vi "Billard2020.vi"(11 "Path":path) -> (0 "Error out":errorcluster)   [LabVIEW 2019]
doc: "Billard2020.vi\n-Call Get_Box or Get_Box_No_Loop, then Call_C, then Draw_Line, then Save_to_Matlab and finally run Analyse.m. \n-To run this VI you have to provide the path of the desired sequence.\n-You can choose before runing if you want to create a ScoreSheet.\n-You can also personalize ScoreSheet.pdf with Band Touch, Ball Touch and Line (as described in the context help of Save_to_Matlab) and choose the detection method of the Billard box (with or without loop).\n-If an error occurs you can get more information about the error by consulting the PDF docsumentation or on : \nhttp://zone.ni.com/reference/fr-XX/help/371361R-0114/lverror/misc_lv_error_codes/"
panel:
  in  "Dark Blue Frame":T1={"Rmax"=14.0, "Rmin"=0.0, "Gmax"=42.0, "Gmin"=0.0, "Bmax"=126.0, "Bmin"=121.0}
  in  "Get Box Whithout Loop":bool
  in  "Parameters":T2={"RedBall"={"Rmin"=160.0, "Rmax"=255.0, "Gmin"=0.0, "Gmax"=160.0, "Bmin"=0.0, "Bmax"=160.0}, "YellowBall"={"Rmin"=140.0, "Rmax"=255.0, "Gmin"=140.0, "Gmax"=255.0, "Bmin"=0.0, "Bmax"=175.0}, "WhiteBall"={"Rmin"=100.0, "Rmax"=255.0, "Gmin"=100.0, "Gmax"=255.0, "Bmin"=100.0, "Bmax"=255.0}, "BlueBG"={"Rmin"=39.0, "Rmax"=62.0, "Gmin"=91.0, "Gmax"=116.0, "Bmin"=202.0, "Bmax"=255.0}, "BallDiameter"=11.0}
  in  "Line":string=".-"
  in  "Ball Touch":u32(colorbox)=1238015
  in  "Band Touch":u32(colorbox)=6618880
  in  "Create Matlab Score Sheet":bool=TRUE
  out "?":picture
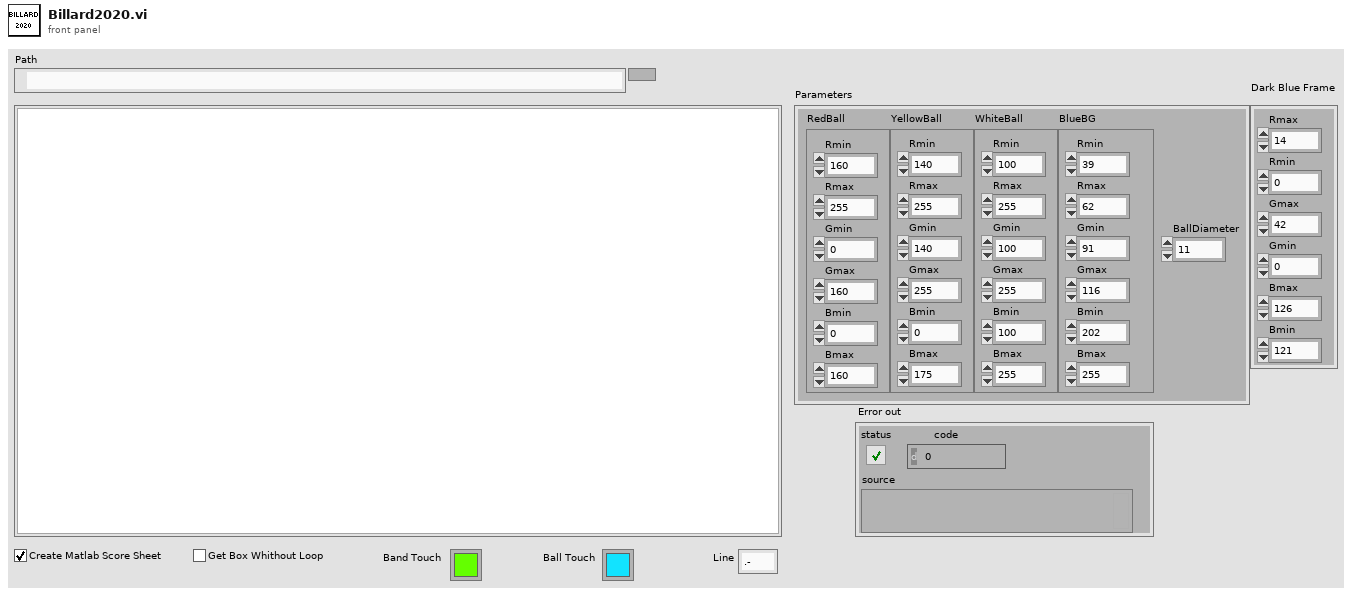
[diagram p1: front panel]
types:
  T1 = cluster{"Rmax":dbl, "Rmin":dbl, "Gmax":dbl, "Gmin":dbl, "Bmax":dbl, "Bmin":dbl}
  T2 = cluster{"RedBall":cluster{"Rmin":dbl, "Rmax":dbl, "Gmin":dbl, "Gmax":dbl, "Bmin":dbl, "Bmax":dbl}, "YellowBall":cluster{"Rmin":dbl, "Rmax":dbl, "Gmin":dbl, "Gmax":dbl, "Bmin":dbl, "Bmax":dbl}, "WhiteBall":cluster{"Rmin":dbl, "Rmax":dbl, "Gmin":dbl, "Gmax":dbl, "Bmin":dbl, "Bmax":dbl}, "BlueBG":cluster{"Rmin":dbl, "Rmax":dbl, "Gmin":dbl, "Gmax":dbl, "Bmin":dbl, "Bmax":dbl}, "BallDiameter":dbl}
  T3 = cluster{"Red":cluster{"X":dbl, "Y":dbl, "Score":dbl}, "Yellow":cluster{"X":dbl, "Y":dbl, "Score":dbl}, "White":cluster{"X":dbl, "Y":dbl, "Score":dbl}}[]
  T4 = cluster{"Ymin":dbl, " Ymax":dbl, "Xmin":dbl, "Xmax":dbl}
  T5 = cluster{"Red":cluster{"X":dbl, "Y":dbl, "Score":dbl}, "Yellow":cluster{"X":dbl, "Y":dbl, "Score":dbl}, "White":cluster{"X":dbl, "Y":dbl, "Score":dbl}}
  T6 = typedef "imagedata.ctl" = cluster{"image type":i32, "image depth":i32, "image":u8[], "mask":u8[], "colors":u32[], "Rectangle":cluster{"left":i16, "top":i16, "right":i16, "bottom":i16}}
  T7 = cluster{dbl[], dbl[], dbl[], dbl[], dbl[], dbl[]}
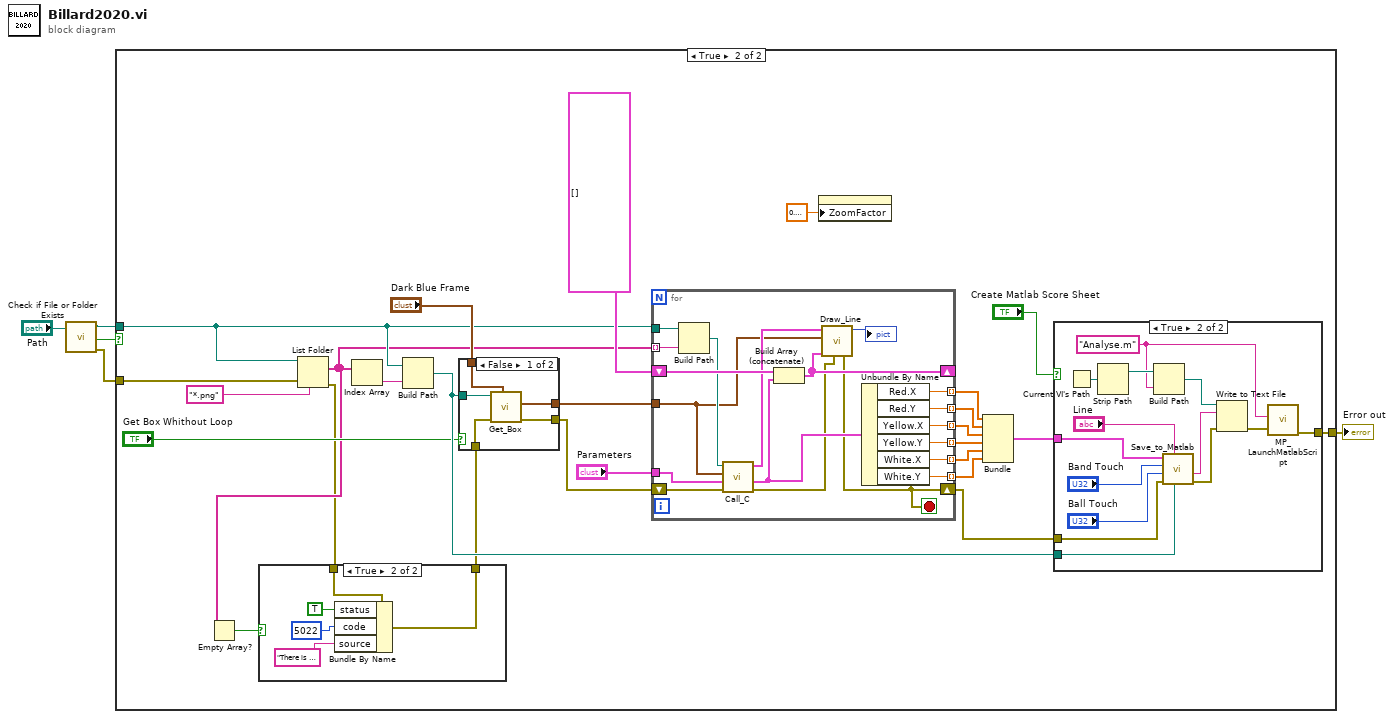
[diagram p0: block diagram]
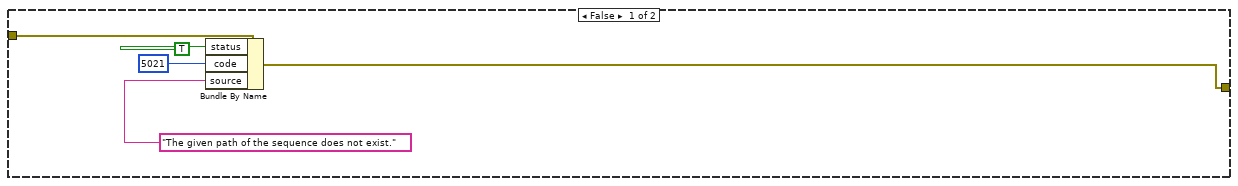
[diagram p2: hidden frame]
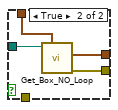
[diagram p4: hidden frame]
diagram:
  n1 = call <vilib>:"Check if File or Folder Exists.vi"("path"="Path") -> ("error out"=w1:errorcluster, "file or folder exists?"=w2:bool, "dup path"=w3:path)  [unwired: 8 in]
  n2 = case shown="True" w2 {
    tunnel: [w6 w27] -> w5
    tunnel: w3 -> [_ w16]
    tunnel: w1 -> [w10 w15]
    frame False {
      n3 = Bundle By Name(cluster=w10, "status"=TRUE, "code"=5021, "source"="The given path of the sequence does not exist.") -> (w6:errorcluster)
    }
    frame True {
      n4 = List Folder(path=w16, pattern="*.png", error in=w15) -> (filenames=w13:string[], error out=w12:errorcluster)  [unwired: 1 in, 2 out]
      n5 = Empty Array?(array=w13) -> (empty?=w14:bool)
      n6 = case shown="True" w14 {
        tunnel: w12 -> [w37 w39]
        tunnel: [w37 w38] -> w11
        frame False {
        }
        frame True {
          n7 = Bundle By Name(cluster=w39, "status"=TRUE, "code"=5022, "source"="There is no png file in the sequence provided.") -> (w38:errorcluster)
        }
      }
      n8 = Index Array(array=w13) -> (element=w35:string)  [unwired: 1 in]
      n9 = Build Path(base path=w16, name or relative path=w35) -> (appended path=w24:path)
      n10 = case shown="False" "Get Box Whithout Loop" {
        tunnel: w24 -> [w47 w51]
        tunnel: "Dark Blue Frame" -> [w46 w48]
        tunnel: [w45 w49] -> w22
        tunnel: [w44 w50] -> w21
        tunnel: w11 -> [w43 _]
        frame False {
          n11 = call "Get_Box.vi"("Dark Blue \nFrame"=w46, "Error in (no error)"=w43, "Path to PNG file"=w47) -> ("Error out"=w44:errorcluster, "BillardBox"=w45:T4)  [unwired: 7 in]
        }
        frame True {
          n12 = call "Get_Box_NO_Loop.vi"("Dark Blue \nFrame"=w48, "Path to PNG file"=w51) -> ("Error out"=w50:errorcluster, "BillardBox"=w49:T4)  [unwired: 8 in]
        }
      }
      n13 = for {
        tunnel: w16 -> [w85]
        tunnel: w13 -> [w84] mode=indexing
        shift-right: [w67] -> w23
        shift-left: w21 -> [w83]
        shift-right: [w79] -> _
        shift-left: T3 [] -> [w82]
        tunnel: [w77] -> w34 mode=indexing
        tunnel: [w76] -> w33 mode=indexing
        tunnel: [w75] -> w32 mode=indexing
        tunnel: [w74] -> w31 mode=indexing
        tunnel: [w73] -> w30 mode=indexing
        tunnel: [w72] -> w29 mode=indexing
        tunnel: "Parameters" -> [w70]
        tunnel: w22 -> [w69]
        stop <- w67 stop-if-true
        n14 = Build Path(base path=w85, name or relative path=w84) -> (appended path=w71:path)
        n15 = call "Call_C.vi"("Error in (no error)"=w83, "Parameters"=w70, "BillardBox"=w69, "Path to PNG file"=w71) -> ("Error out"=w68:errorcluster, "Balls coordinates"=w78:T5, "Image data"=w81:T6)  [unwired: 5 in]
        n16 = Build Array (concatenate)(w82, w78) -> (w79:T3)
        n17 = call "Draw_Line.vi"("Error in (no error)"=w68, "All balls \ncoordinates"=w79, "BillardBox"=w69, "Image data"=w81) -> ("New picture"=→"?":picture, "Error out"=w67:errorcluster)  [unwired: 6 in]
        n18 = Unbundle By Name(w78) -> ("Red.X"=w77:dbl, "Red.Y"=w76:dbl, "Yellow.X"=w75:dbl, "Yellow.Y"=w74:dbl, "White.X"=w73:dbl, "White.Y"=w72:dbl)
      }
      n19 = property class="Pict"("ZoomFactor"=sgl 0.9 ("Zoom Factor")) -> ()  [unwired: 2 in, 2 out]
      n20 = Bundle(w34, w33, w32, w31, w30, w29) -> (w25:T7)  [unwired: 1 in]
      n21 = case shown="True" "Create Matlab Score Sheet" {
        tunnel: [w52 w61] -> w27
        tunnel: w25 -> [_ w58]
        tunnel: w24 -> [_ w57]
        tunnel: w23 -> [w52 w54]
        frame False {
        }
        frame True {
          w62 = "Analyse.m" ("name or relative path")
          n22 = Current VI's Path() -> (path=w64:path)
          n23 = Strip Path(path=w64) -> (stripped path=w63:path)  [unwired: 1 out]
          n24 = Build Path(base path=w63, name or relative path=w62) -> (appended path=w66:path)
          n25 = call "Save_to_Matlab.vi"("Path to PNG file"=w57, "Line"="Line", "Error in \n(no error)"=w54, "Ball Touch"="Ball Touch", "Band Touch"="Band Touch", "Balls coordinates"=w58) -> ("Error out"=w53:errorcluster, "Script of Analyse.m"=w60:string)  [unwired: 4 in]
          n26 = Write to Text File(file (use dialog)=w66, text=w60, error in=w53) -> (error out=w65:errorcluster)  [unwired: 1 in, 2 out]
          n27 = call "MP_LaunchMatlabScript.vi"("error in (no error)"=w65, "matlab script name with extension"=w62) -> ("error out"=w61:errorcluster)  [unwired: 5 in, 4 out]
        }
      }
    }
  }
  "Error out" <- w5
